vi "WithParent_ReturnsParentTag.vi"() -> (0 "error out":errorcluster)   [LabVIEW 2017, in "ResultTree.Tests.lvlib" / "GetParent.lvlib"]
uses:
  GetParent.lvlib
  2a6c7ef5-d8ea-4de4-ba7d-c6663dbf2225.vi
  Constraint/IsEqual/Create.vi
  Constraint/IsEqual/IsEqual.lvclass
  ResultTree/ResultTree.lvclass
panel:
  in  "Tree":string(tree)
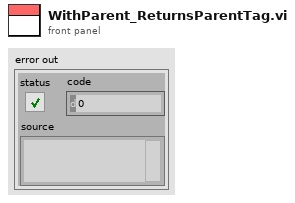
[diagram p1: front panel]
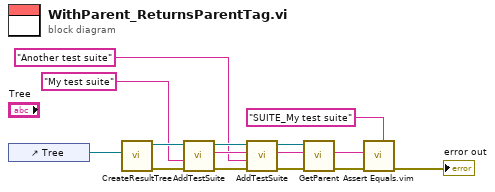
[diagram p0: block diagram]
diagram:
  n1 = control-ref of="Tree"() -> (w14:refnum<vi>)
  n2 = call "CreateResultTree.vi"("Tree Refnum"=w14) -> ("error out"=w13:errorcluster, "ResultTree out"=w12:refnum<class "ResultTree.lvclass">)  [unwired: 9 in]
  n3 = call "AddTestSuite.vi"("error in (no error)"=w13, "Name"="My test suite", "ResultTree in"=w12) -> ("error out"=w9:errorcluster, "Tag Name"=w7:string, "ResultTree out"=w10:refnum<class "ResultTree.lvclass">)  [unwired: 6 in]
  n4 = call "AddTestSuite.vi"("error in (no error)"=w9, "Name"="Another test suite", "Parent Tag (\"\")"=w7, "ResultTree in"=w10) -> ("error out"=w8:errorcluster, "Tag Name"=w3:string, "ResultTree out"=w4:refnum<class "ResultTree.lvclass">)  [unwired: 5 in]
  n5 = call "GetParent.vi"("error in (no error)"=w8, "Tag"=w3, "ResultTree in"=w4) -> ("error out"=w2:errorcluster, "Parent Tag"=w1:string)  [unwired: 6 in, 1 out]
  n6 = call "Assert Equals.vim"("Expected"="SUITE_My test suite" ("Name"), "error in (no error)"=w2, "Actual"=w1) -> ("error out"=→"error out":errorcluster)  [unwired: 8 in]
